vi "valvesAdam'sEmpireExpands.vi"() -> ()   [LabVIEW 2016]
uses:
  <vilib>/DAQmx/write.llb/DAQmx Write (Digital 1D Bool NChan 1Samp 1Line).vi
  <vilib>/DAQmx/read.llb/DAQmx Read (Analog 1D DBL NChan 1Samp).vi
  <vilib>/DAQmx/create/channels.llb/DAQmx Create Channel (AI-Voltage-Basic).vi
  <vilib>/DAQmx/create/channels.llb/DAQmx Create Channel (DO-Digital Output).vi
  <vilib>/DAQmx/miscellaneous.llb/DAQmx Fill In Error Info.vi
panel:
  out "Scroll Pump Pressure 2 (mbar)":dbl format="%.2f"
  out "Chamber Pressure 2 (mbar)":dbl format="%.2f"
  out "Scroll Pump Pressure (mBar)":string
  out "Chamber Pressure (mBar)":string
  out "Gate Valve Open":bool
  out "Gate Valve Closed":bool
  in  "Pump Valve":bool
  in  "Gate Valve":bool
  in  "Roughing Valve":bool
  in  "stop":bool
  # "Turbo Pump"
  # "Scroll (Roughing) Pump"
  # "Back\nPressure\nReadout"
  # "Chamber\nPressure\nReadout"
  # "Chamber"
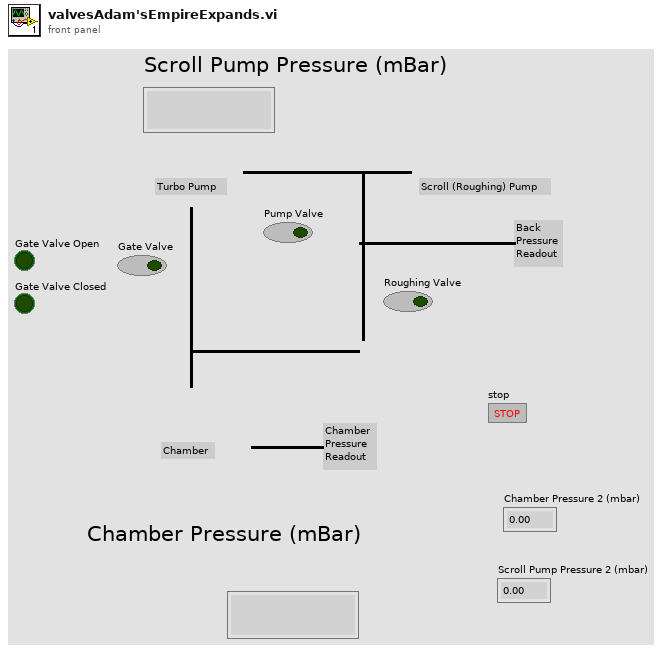
[diagram p1: front panel]
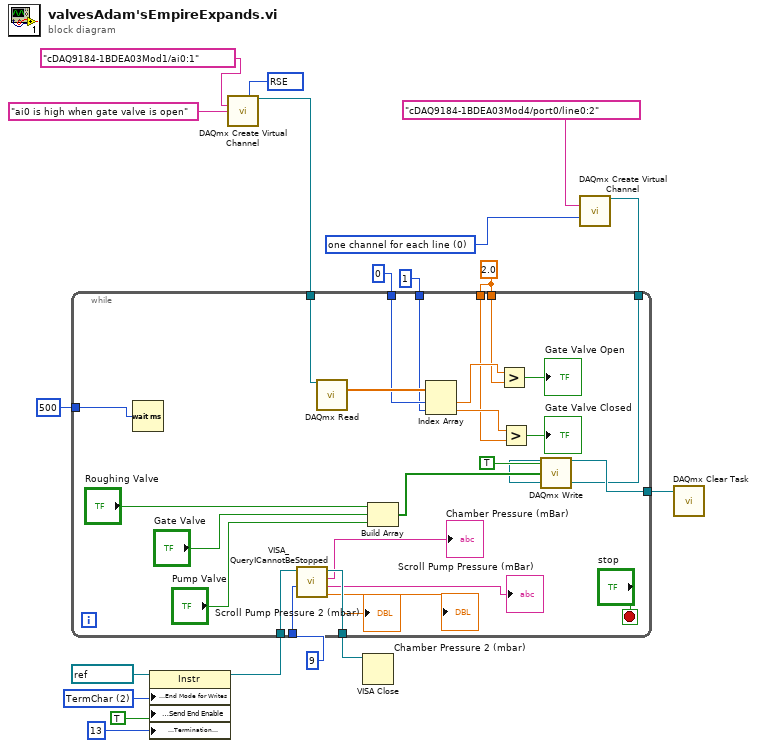
[diagram p0: block diagram]
diagram:
  w3 = 2.0 ("y")
  w11 = 0 items=["one channel for each line", "one channel for all lines"] ("line grouping")
  w15 = 10083 items=["Default"=-1, "RSE"=10083, "NRSE"=10078, "Differential"=10106, "Pseudodifferential"=12529] ("input terminal configuration")
  w18 = u16 2 items=["None", "Last Bit", "TermChar", "Break"] ("Serial Settings:End Mode for Writes")
  n1 = property class="Instr"(reference=refnum<visa-resource-name> "COM8" ("VISA resource name"), "Serial Settings:End Mode for Writes"=w18, "Message Based Settings:Send End Enable"=TRUE, "Message Based Settings:Termination Character"=u8 13) -> (reference out=w7:refnum<visa-resource-name>)  [unwired: 1 in, 1 out]
  n2 = call-poly <vilib>:"DAQmx Create Virtual Channel.vi"("input terminal configuration"=w15, "physical channels"=tag "cDAQ9184-1BDEA03Mod1/ai0:1" ("lines"), "name to assign"="ai0 is high when gate valve is open") -> ("task out"=w12:refnum<k21>)  [unwired: 11 in, 1 out]
  n3 = call-poly <vilib>:"DAQmx Create Virtual Channel.vi"("lines"=tag "cDAQ9184-1BDEA03Mod4/port0/line0:2", "line grouping"=w11) -> ("task out"=w8:refnum<k21>)  [unwired: 12 in, 1 out]
  n4 = while {
    tunnel: w12 -> [w36]
    tunnel: [w33] -> w9
    tunnel: w8 -> [w32]
    tunnel: w7 -> [w31]
    tunnel: 9 -> [w30]
    tunnel: [w29] -> w5
    tunnel: u32 500 ("milliseconds to wait") -> [w26]
    tunnel: w3 -> [w25]
    tunnel: w3 -> [w24]
    tunnel: 0 ("index") -> [w23]
    tunnel: 1 ("index") -> [w22]
    stop <- "stop" stop-if-true
    n5 = Wait (ms)(milliseconds to wait=w26) -> ()  [unwired: 1 out]
    n6 = call "VISA_QueryICannotBeStopped.vi"("Numeric"=w30, "VISA Refnum in"=w31) -> ("Chamber Pressure 2 (mbar)"=→"Chamber Pressure 2 (mbar)":dbl, "Scroll Pump Pressure (mBar)"=→"Scroll Pump Pressure (mBar)":string, "Chamber Pressure (mBar)"=→"Chamber Pressure (mBar)":string, "VISA Refnum out"=w29:refnum<visa-resource-name>, "Scroll Pump Pressure 2 (mbar)"=→"Scroll Pump Pressure 2 (mbar)":dbl)  [unwired: 5 in]
    n7 = call-poly <vilib>:"DAQmx Read.vi"("task/channels in"=w36) -> ("data"=w41:dbl[])  [unwired: 12 in, 2 out]
    n8 = Build Array("Roughing Valve", "Gate Valve", "Pump Valve") -> (w34:bool[])
    n9 = Index Array(array=w41, index #1=w23, index #2=w22) -> (element #1=w40:dbl, element #2=w38:dbl)
    n10 = Greater?(x=w40, y=w25) -> (0:→"Gate Valve Open":bool)
    n11 = Greater?(x=w38, y=w24) -> (0:→"Gate Valve Closed":bool)
    n12 = call-poly <vilib>:"DAQmx Write.vi"("task/channels in"=w32, "auto start"=TRUE, "data"=w34) -> ("task out"=w33:refnum<k21>)  [unwired: 10 in, 2 out]
  }
  n13 = VISA Close(VISA resource name=w5) -> ()  [unwired: 1 in, 1 out]
  n14 = call <vilib>:"DAQmx Clear Task.vi"("task in"=w9) -> ()  [unwired: 14 in, 1 out]
